vi "Set Image.vi"(8 "error in (no error)":errorcluster, 10 "Picture":picture, 11 "VI Reference Control in":refnum<class "VI Reference Control.lvclass">) -> (0 "error out":errorcluster, 3 "VI Reference Control out":refnum<class "VI Reference Control.lvclass">)   [LabVIEW 2016, in "VI Reference Control.lvclass"]
uses:
  VI Reference Control.lvclass
  VI Reference Control.lvclass/VI Reference Control.ctl
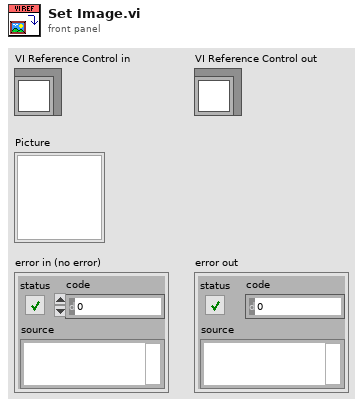
[diagram p1: front panel]
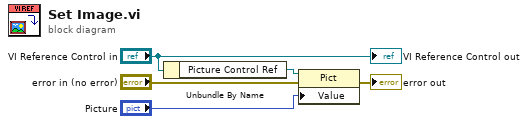
[diagram p0: block diagram]
diagram:
  n1 = Unbundle By Name("VI Reference Control in") -> ("Picture Control Ref"=w2:refnum<vi>)
  n2 = property on="Property Node" class="Pict"(reference=w2, error in="error in (no error)", "Value"="Picture") -> (error out=→"error out":errorcluster)  [unwired: 1 out]
  "VI Reference Control out" <- "VI Reference Control in"
